vi "Day 11-2.vi"() -> ()   [LabVIEW 2019, in "Day 11.lvlib"]
uses:
  Day 11.lvlib
panel:
  out "Step":i32
  out "Array n":i32[][](array[numeric])=[[1, 1, 1, 3, 2, 2, 7, 5, 4, 8], [1, 1, 5, 3, 2, 2, 2, 6, 4, 4], [1, 6, 3, 2, 2, 2, 3, 8, 5, 4], [1, 5, 2, 2, 2, 3, 5, 1, 8, 6], [1, 5, 2, 2, 3, 5, 1, 1, 1, 1], [1, 4, 2, 3, 5, 1, 1, 1, 1, 1], [3, 4, 4, 6, 1, 1, 1, 1, 1, 1], [9, 9, 1, 2, 3, 3, 2, 1, 1, 7], [8, 1, 2, 4, 0, 0, 4, 2, 7, 5], [7, 1, 2, 0, 0, 0, 0, 7, 5, 4]]
  out "Ligths":bool[][](array[boolean])=[[FALSE, FALSE, FALSE, FALSE, FALSE, FALSE, FALSE, FALSE, FALSE, FALSE], [FALSE, FALSE, FALSE, FALSE, FALSE, FALSE, FALSE, FALSE, FALSE, FALSE], [FALSE, FALSE, FALSE, FALSE, FALSE, FALSE, FALSE, FALSE, FALSE, FALSE], [FALSE, FALSE, FALSE, FALSE, FALSE, FALSE, FALSE, FALSE, FALSE, FALSE], [FALSE, FALSE, FALSE, FALSE, FALSE, FALSE, FALSE, FALSE, FALSE, FALSE], [FALSE, FALSE, FALSE, FALSE, FALSE, FALSE, FALSE, FALSE, FALSE, FALSE], [FALSE, FALSE, FALSE, FALSE, FALSE, FALSE, FALSE, FALSE, FALSE, FALSE], [FALSE, FALSE, FALSE, FALSE, FALSE, FALSE, FALSE, FALSE, FALSE, FALSE], [FALSE, FALSE, FALSE, FALSE, TRUE, TRUE, FALSE, FALSE, FALSE, FALSE], [FALSE, FALSE, FALSE, TRUE, TRUE, TRUE, TRUE, FALSE, FALSE, FALSE]]
  out "Flashes":i32=1683
  out "Array n-1":i32[][](array[numeric])=[[0, 0, 0, 2, 1, 1, 6, 4, 3, 7], [0, 0, 4, 2, 1, 1, 1, 5, 3, 3], [0, 5, 2, 1, 1, 1, 2, 7, 4, 3], [0, 4, 1, 1, 1, 2, 4, 0, 7, 5], [0, 4, 1, 1, 2, 4, 0, 0, 0, 0], [0, 3, 1, 2, 4, 0, 0, 0, 0, 0], [2, 3, 3, 5, 0, 0, 0, 0, 0, 0], [8, 8, 0, 0, 0, 0, 0, 0, 0, 6], [7, 0, 0, 0, 9, 9, 0, 0, 6, 4], [6, 0, 0, 8, 6, 6, 8, 5, 4, 3]]
  in  "String":string="8826876714\n3127787238\n8182852861\n4655371483\n3864551365\n1878253581\n8317422437\n1517254266\n2621124761\n3473331514"
  # "1671\ntoo low"
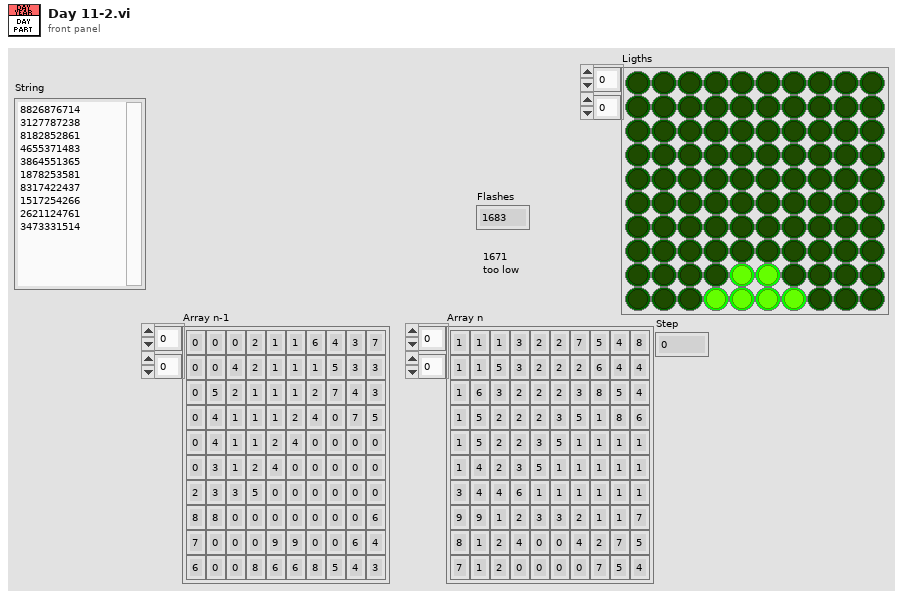
[diagram p1: front panel]
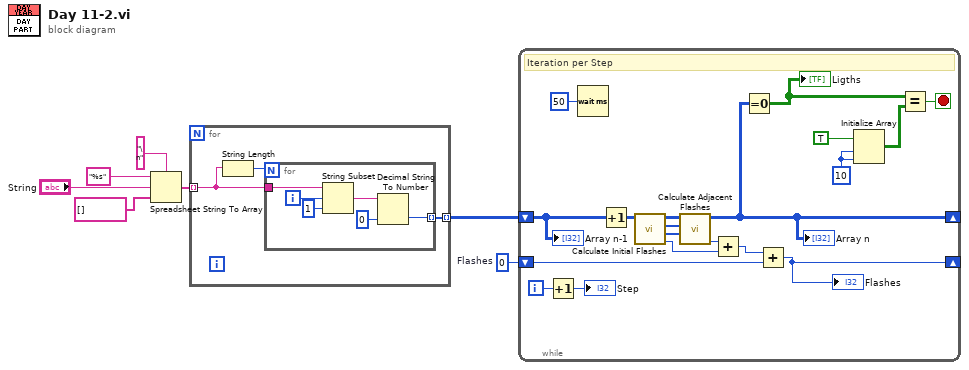
[diagram p0: block diagram]
diagram:
  w1 = 0  # Flashes
  n1 = Spreadsheet String To Array(delimiter (Tab)="\n", format string="%s", spreadsheet string="String", array type (2D Dbl)=string[] []) -> (array=w3:string[])
  n2 = for {
    tunnel: w3 -> [w10] mode=indexing
    tunnel: [w8] -> w2 mode=indexing
    n3 = String Length(string=w10) -> (length=w9:i32)
    n4 = for {
      N: w9 -> [_]
      tunnel: w10 -> [w16]
      tunnel: [w12] -> w8 mode=indexing
      i -> [w15]
      n5 = String Subset(string=w16, offset (0)=w15, length (rest)=1 ("length (rest)")) -> (substring=w13:string)
      n6 = Decimal String To Number(string=w13, default (0L)=0 ("default (0 I32)")) -> (number=w12:i32)  [unwired: 1 in, 1 out]
    }
  }
  n7 = while {
    shift-right: [w25] -> _
    shift-left: w2 -> [w26]
    shift-right: [w24] -> _
    shift-left: w1 -> [w28]
    i -> [w18]
    stop <- w19 stop-if-true
    w22 = 10 ("dimension size")
    # "Iteration per Step"
    n8 = Increment(x=w18) -> (x+1=→"Step":i32)
    n9 = Wait (ms)(milliseconds to wait=u32 50) -> ()  [unwired: 1 out]
    n10 = Increment(x=w26) -> (x+1=w35:i32[][])
    n11 = call "Calculate Initial Flashes.vi"("Octopus Energy Matrix In"=w35) -> ("Flash Count"=w30:i32, "Flashes Columns"=w32:i32[], "Flashes Rows"=w33:i32[], "Octopus Energy Matrix Out"=w34:i32[][])  [unwired: 7 in]
    n12 = call "Calculate Adjacent Flashes.vi"("Flashes Columns"=w32, "Flashes Rows"=w33, "Octopus Energy Matrix In"=w34) -> ("Flash Count"=w31:i32, "Octopus Energy Matrix Out"=w25:i32[][])  [unwired: 7 in]
    "Array n" <- w25
    n13 = Add(x=w31, y=w30) -> (x+y=w29:i32)
    n14 = Equal To 0?(x=w25) -> (x = 0?=w21:bool[][])
    "Ligths" <- w21
    n15 = Add(x=w29, y=w28) -> (x+y=w24:i32)
    "Flashes" <- w24
    n16 = Initialize Array(TRUE, w22, w22) -> (w20:bool[][])
    n17 = Equal?(x=w21, y=w20) -> (x = y?=w19:bool)
    "Array n-1" <- w26
  }
